vi "varlongitude.vi"() -> ()   [LabVIEW 2012]
panel:
  out "longitude":i32
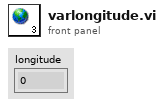
[diagram p1: front panel]
diagram:
